vi "Preallocate Method Results.vi"(9 "Test Methods":string[](array[string]), 10 "Test Case":string) -> (3 "Test Case Result out":T1)   [LabVIEW 2020, in "Test Case Result.lvlib"]
uses:
  Test Case Result.lvlib
  Test Case Result.ctl
  Method Result/Method Result.ctl
  Assertion Result/Public/TypeDefs/Status.ctl
  Assertion Result/Assertion Result.ctl
  Assertion Result/Public/TypeDefs/Assertion Type.ctl
  Assertion Result/Assertion Result.lvlib
  Method Result/Method Result.lvlib
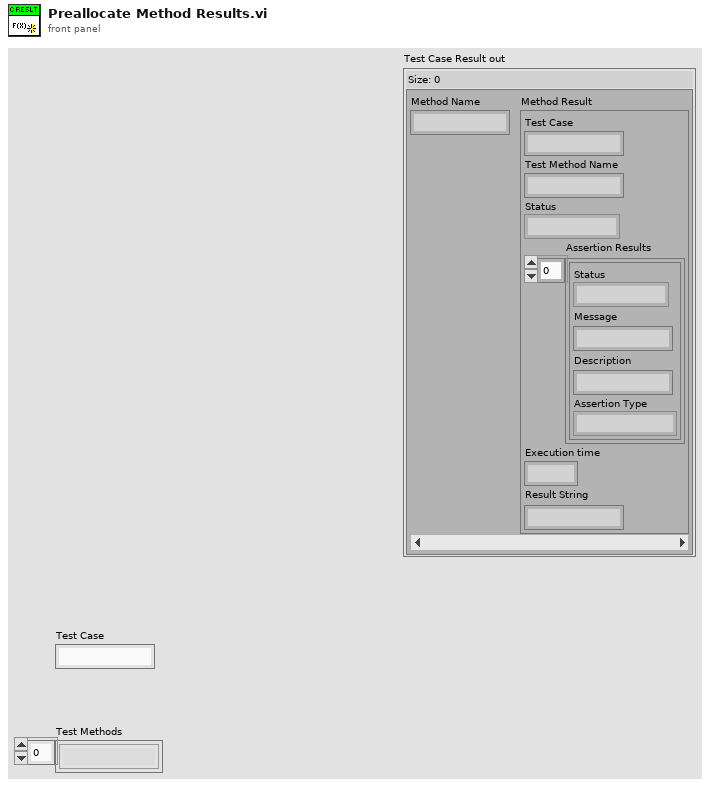
[diagram p1: front panel]
types:
  T1 = typedef "Test Case Result.lvlib/Test Case Result.ctl" = map{string, T2}
  T2 = typedef "Method Result.lvlib/Method Result.ctl" = cluster{"Test Case":string, "Test Method Name":string, "Status":T3, "Assertion Results":T4[], "Execution time":dbl, "Result String":string}
  T3 = typedef "Assertion Result.lvlib/Status.ctl" = enum16{"Pass", "Fail", "Error", "Skipped", "Setup Error", "Broken", "Teardown Error"}
  T4 = typedef "Assertion Result.lvlib/Assertion Result.ctl" = cluster{"Status":T3, "Message":string, "Description":string, "Assertion Type":T5}
  T5 = typedef "Assertion Result.lvlib/Assertion Type.ctl" = enum16{"None", "Pass", "Fail", "Skip", "Pass if Equal", "Fail if Equal", "Pass if Error", "Fail if Error", "Pass if", "Fail if"}
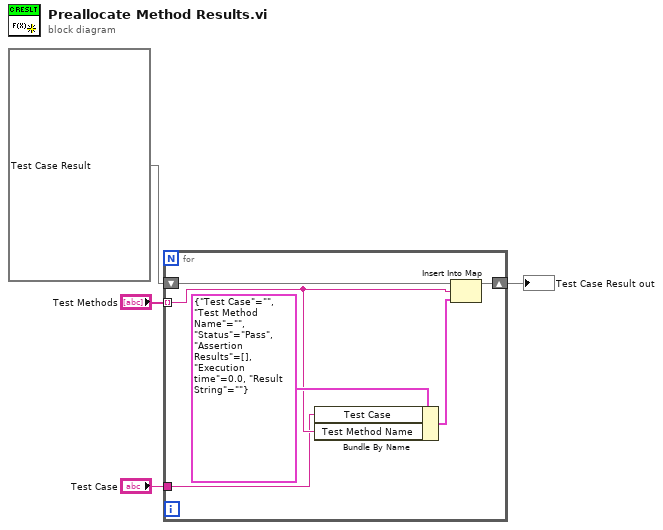
[diagram p0: block diagram]
diagram:
  n1 = for {
    shift-right: [w9] -> w2
    shift-left: T1 {} ("Test Case Result in") -> [w10]
    tunnel: "Test Methods" -> [w7] mode=indexing
    tunnel: "Test Case" -> [w6]
    n2 = Bundle By Name(cluster=T2 {"Test Case"="", "Test Method Name"="", "Status"=enum."Pass", "Assertion Results"=[], "Execution time"=0.0, "Result String"=""} ("Cluster of class private data"), "Test Case"=w6, "Test Method Name"=w7) -> (w5:T2)
    n3 = Insert Into Map(map in=w10, key=w7, value=w5) -> (map out=w9:T1)  [unwired: 2 out]
  }
  "Test Case Result out" <- w2
